vi "SpecPage.vi"(10 "Spec Page Interface":T1, 11 "MetaDataObj in":refnum<class "MetaDataObj.lvclass">) -> (3 "MetaDataObj out":refnum<class "MetaDataObj.lvclass">)   [LabVIEW 2016, in "MeasurementMetaData.lvclass"]
uses:
  MeasurementMetaData.lvclass
  <resource>/dialog/NewProjectWizard/Spec Page Interface.ctl
  <resource>/dialog/NewProjectWizard/MetaDataObj/MetaDataObj.lvclass
  UI References Type Definition.ctl
  C:/Program Files (x86)/National Instruments/LabVIEW 2016/resource/dialog/NewProjectWizard/MetaDataObj/MetaDataObj.lvclass
  MeasurementMetaData.lvclass/MeasurementMetaData.ctl
  <resource>/dialog/NewProjectWizard/MetaDataObj/MetaDataObj.lvclass/MetaDataObj.ctl
  Plugin Settings.ctl
  <resource>/dialog/NewProjectWizard/MetaDataObj/Accessors/Write Project Root.vi
  <resource>/dialog/NewProjectWizard/MetaDataObj/Accessors/Write Project Name.vi
  <resource>/dialog/NewProjectWizard/MetaDataObj/Accessors/Write File Prefix.vi
panel:
  in  "Project Name":string
  in  "Project Root":path
  in  "Measurement Name":string="New Measurement"
  in  "Acquisition Mode":enum16{"Continuous", "Single-Shot"}(ring)=enum."Single-Shot"
  in  "PSU?":bool
  in  "FGEN?":bool
  in  "Scope?":bool
  in  "DMM?":bool
  in  "Override Close Method":bool
  in  "Override Measure Method":bool
  in  "Override Configure Method":bool
  in  "Generate Custom Results Object":bool
  # "Select Methods to Override"
  # "Select Required Hardware"
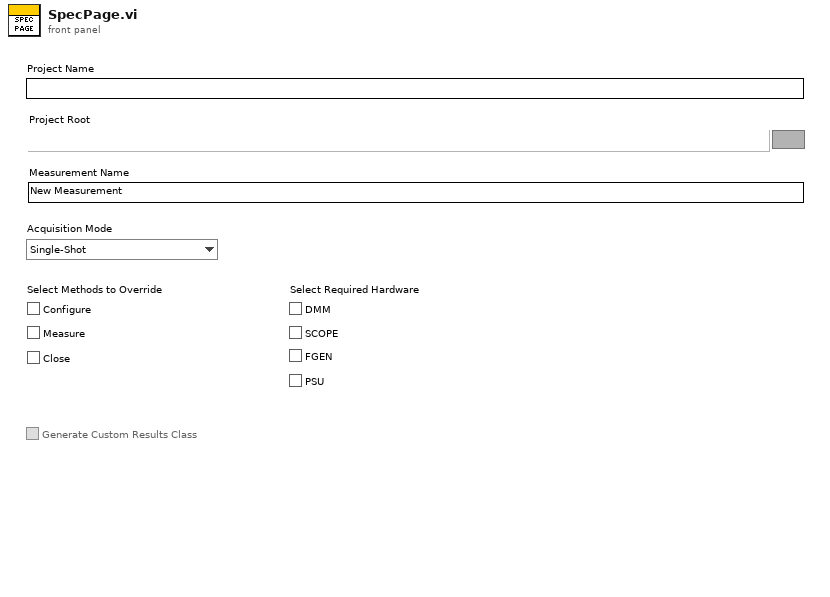
[diagram p1: front panel]
types:
  T1 = typedef "Spec Page Interface.ctl" = cluster{"\"Tab Forward To\" Refnum":refnum<vi>, "\"Tab Backward To\" Refnum":refnum<vi>, "Errors":refnum<user-event>, "Quit":refnum<user-event>}
  T2 = typedef "MeasurementMetaData.lvclass/UI References Type Definition.ctl" = cluster{"Measurement Name":refnum<vi>, "Project Name":refnum<vi>, "Project Root":refnum<vi>, "PSU?":refnum<vi>, "FGEN?":refnum<vi>, "Scope?":refnum<vi>, "DMM?":refnum<vi>, "Override Close Method":refnum<vi>, "Override Measure Method":refnum<vi>, "Generate Custom Results Object":refnum<vi>, "Override Configure Method":refnum<vi>, "Acquisition Mode":refnum<vi>}
  T3 = typedef "MeasurementMetaData.lvclass/Plugin Settings.ctl" = cluster{"Override Configure Method":bool, "Generate Custom Results Object":bool, "Override Measure Method":bool, "Override Close Method":bool, "Scope?":bool, "DMM?":bool, "FGEN?":bool, "PSU?":bool, "Acquisition Mode":enum16{"Continuous", "Single-Shot"}}
  T4 = enum8{"Enabled", "Disabled", "Disabled and Grayed Out"}
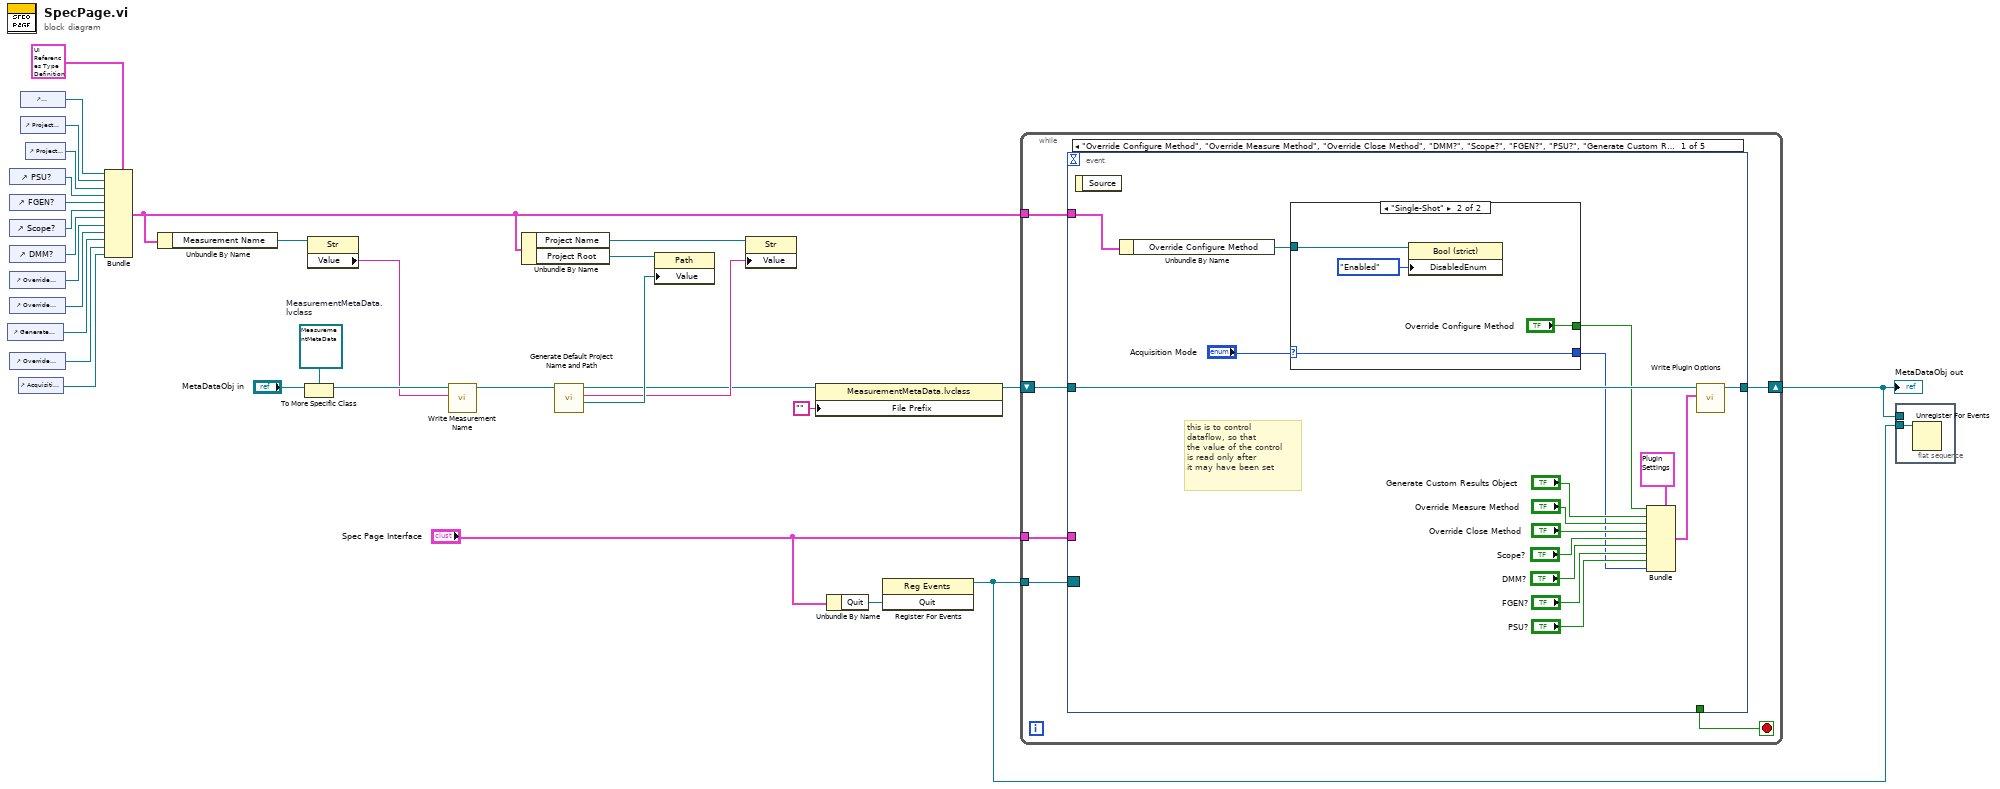
[diagram p0: block diagram]
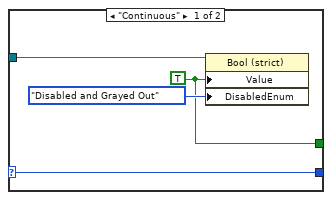
[diagram p2: hidden frame]
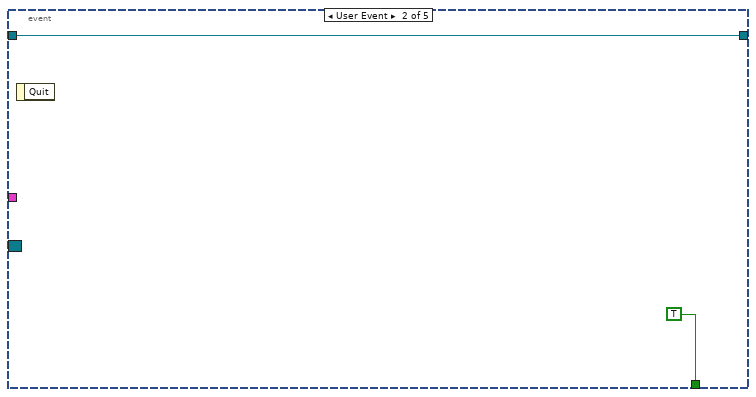
[diagram p3: hidden frame]
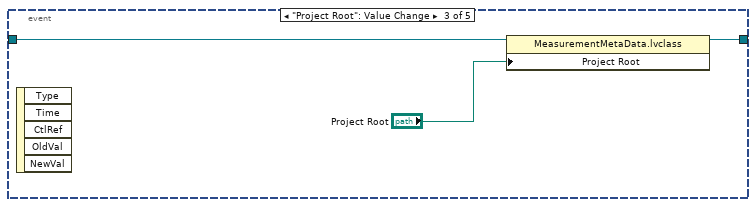
[diagram p4: hidden frame]
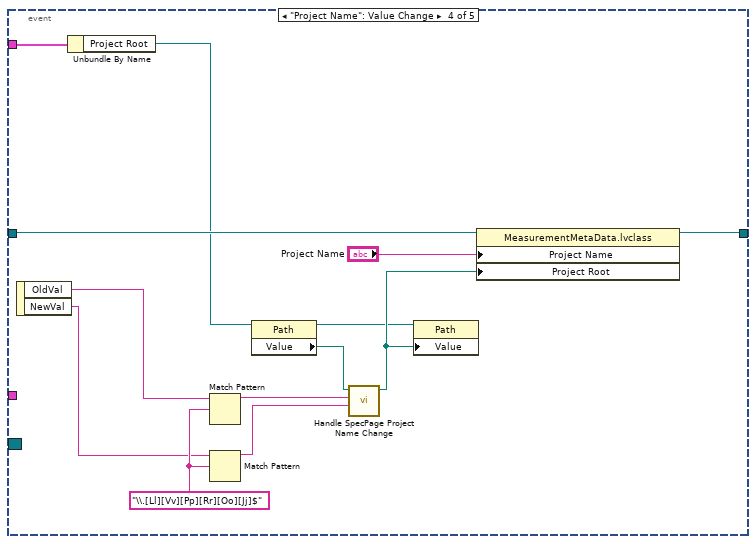
[diagram p5: hidden frame]
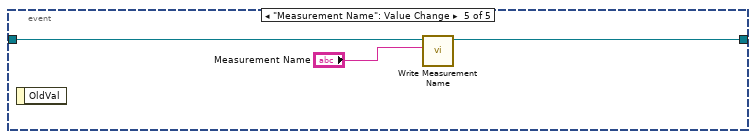
[diagram p6: hidden frame]
diagram:
  w17 = refnum<class "MeasurementMetaData.lvclass"> refnum  # MeasurementMetaData.lvclass
  n1 = control-ref of="Generate Custom Results Object"() -> (w3:refnum<vi>)
  n2 = control-ref of="PSU?"() -> (w25:refnum<vi>)
  n3 = control-ref of="FGEN?"() -> (w24:refnum<vi>)
  n4 = control-ref of="Scope?"() -> (w23:refnum<vi>)
  n5 = control-ref of="DMM?"() -> (w22:refnum<vi>)
  n6 = control-ref of="Override Close Method"() -> (w21:refnum<vi>)
  n7 = control-ref of="Override Measure Method"() -> (w20:refnum<vi>)
  n8 = control-ref of="Override Configure Method"() -> (w1:refnum<vi>)
  n9 = control-ref of="Acquisition Mode"() -> (w2:refnum<vi>)
  n10 = control-ref of="Measurement Name"() -> (w28:refnum<vi>)
  n11 = control-ref of="Project Name"() -> (w27:refnum<vi>)
  n12 = control-ref of="Project Root"() -> (w26:refnum<vi>)
  n13 = Bundle(cluster=T2 {"Measurement Name"=refnum, "Project Name"=refnum, "Project Root"=refnum, "PSU?"=refnum, "FGEN?"=refnum, "Scope?"=refnum, "DMM?"=refnum, "Override Close Method"=refnum, "Override Measure Method"=refnum, "Generate Custom Results Object"=refnum, "Override Configure Method"=refnum, "Acquisition Mode"=refnum} ("output cluster"), "Measurement Name"=w28, "Project Name"=w27, "Project Root"=w26, "PSU?"=w25, "FGEN?"=w24, "Scope?"=w23, "DMM?"=w22, "Override Close Method"=w21, "Override Measure Method"=w20, "Generate Custom Results Object"=w3, "Override Configure Method"=w1, "Acquisition Mode"=w2) -> (w7:T2)
  n14 = Unbundle By Name(w7) -> ("Measurement Name"=w6:refnum<vi>)
  n15 = To More Specific Class(target class=w17, reference="MetaDataObj in") -> (specific class reference=w16:refnum<class "MeasurementMetaData.lvclass">)  [unwired: 1 in, 1 out]
  n16 = property class="Str"(reference=w6) -> ("Value"=w5:string)  [unwired: 1 in, 2 out]
  n17 = call "Write Measurement Name.vi"("Measurement Name"=w5, "MeasurementMetaData in"=w16) -> ("MeasurementMetaData out"=w15:refnum<class "MeasurementMetaData.lvclass">)  [unwired: 8 in, 1 out]
  n18 = Unbundle By Name(w7) -> ("Project Name"=w11:refnum<vi>, "Project Root"=w13:refnum<vi>)
  n19 = call <resource>:"Generate Default Project Name and Path.vi"("DNL_MetaDataObj in"=w15) -> ("Project Root"=w12:path, "Project Name"=w10:string, "DNL_MetaDataObj out"=w4:refnum<class "MeasurementMetaData.lvclass">)  [unwired: 8 in]
  n20 = property class="Path"(reference=w13, "Value"=w12) -> ()  [unwired: 1 in, 2 out]
  n21 = property class="Str"(reference=w11, "Value"=w10) -> ()  [unwired: 1 in, 2 out]
  n22 = property class="MeasurementMetaData.lvclass"(reference=w4, "File Prefix"="") -> (reference out=w8:refnum<class "MeasurementMetaData.lvclass">)  [unwired: 1 in, 1 out]
  n23 = Unbundle By Name("Spec Page Interface") -> ("Quit"=w14:refnum<user-event>)
  n24 = register-events(w14) -> (reference out=w31:refnum<event-registration>)  [unwired: 2 in, 1 out]
  n25 = while {
    tunnel: w31 -> [w35]
    tunnel: w7 -> [w33]
    tunnel: "Spec Page Interface" -> [w32]
    shift-right: [w36] -> w29
    shift-left: w8 -> [w37]
    stop <- w34 stop-if-true
    n26 = event shown="[0] \"Override Configure Method\", \"Override Measure Method\", \"Override Close Method\", \"DMM?\", \"Scope?\", \"FGEN?\", \"PSU?\", \"Generate Custom Results Object\", \"Acquisition Mode\": Value Change" {
      selector: w35 -> [_ _ _ _ _]
      dyn-events: _ -> [_ _ _ _ _]
      timeout: _ -> [_ _ _ _ _]
      tunnel: w37 -> [w49 w62 w65 w79 w81]
      tunnel: [w48 w62 w66 w68 w80] -> w36
      tunnel: [_ TRUE _ _ _] -> w34
      tunnel: w33 -> [w42 _ _ w73 _]
      tunnel: w32 -> [_ _ _ _ _]
      event "Override Configure Method", "Override Measure Method", "Override Close Method", "DMM?", "Scope?", "FGEN?", "PSU?", "Generate Custom Results Object", "Acquisition Mode": Value Change {
        # "this is to control\ndataflow, so that\nthe value of the control\nis read only after\nit may have been set"
        n27 = event-data() -> ()  [unwired: 1 in, 1 out]
        n28 = Unbundle By Name(w42) -> ("Override Configure Method"=w41:refnum<vi>)
        n29 = case shown="\"Single-Shot\"" "Acquisition Mode" {
          selector: "Acquisition Mode" -> [w57 w61]
          tunnel: w41 -> [w56 w60]
          tunnel: [w57 w61] -> w39
          tunnel: [w54 "Override Configure Method"] -> w38
          frame "Continuous" {
            w54 = TRUE ("Value")
            n30 = property class="Bool (strict)"(reference=w56, "Value"=w54, "DisabledEnum"=T4."Disabled and Grayed Out" ("Disabled")) -> ()  [unwired: 1 in, 2 out]
          }
          frame "Single-Shot" {
            n31 = property class="Bool (strict)"(reference=w60, "DisabledEnum"=T4."Enabled" ("Disabled")) -> ()  [unwired: 1 in, 2 out]
          }
        }
        n32 = Bundle(cluster=T3 {"Override Configure Method"=FALSE, "Generate Custom Results Object"=FALSE, "Override Measure Method"=FALSE, "Override Close Method"=FALSE, "Scope?"=FALSE, "DMM?"=FALSE, "FGEN?"=FALSE, "PSU?"=FALSE, "Acquisition Mode"=enum."Continuous"} ("Plugin Options"), "Override Configure Method"=w38, "Generate Custom Results Object"="Generate Custom Results Object", "Override Measure Method"="Override Measure Method", "Override Close Method"="Override Close Method", "Scope?"="Scope?", "DMM?"="DMM?", "FGEN?"="FGEN?", "PSU?"="PSU?", "Acquisition Mode"=w39) -> (w50:T3)
        n33 = call "Write Plugin Options.vi"("Plugin Options"=w50, "MeasurementMetaData in"=w49) -> ("MeasurementMetaData out"=w48:refnum<class "MeasurementMetaData.lvclass">)  [unwired: 8 in, 1 out]
      }
      event User Event {
        n34 = event-data() -> ()  [unwired: 1 in, 1 out]
      }
      event "Project Root": Value Change {
        n35 = event-data() -> ()  [unwired: 1 in, 5 out]
        n36 = property class="MeasurementMetaData.lvclass"(reference=w65, "Project Root"="Project Root") -> (reference out=w66:refnum<class "MeasurementMetaData.lvclass">)  [unwired: 1 in, 1 out]
      }
      event "Project Name": Value Change {
        w78 = "\\.[Ll][Vv][Pp][Rr][Oo][Jj]$" ("regular expression")
        n37 = event-data() -> ("OldVal"=w77:string, "NewVal"=w76:string)  [unwired: 1 in]
        n38 = Unbundle By Name(w73) -> ("Project Root"=w72:refnum<vi>)
        n39 = Match Pattern(string=w77, regular expression=w78) -> (before substring=w74:string)  [unwired: 1 in, 3 out]
        n40 = Match Pattern(string=w76, regular expression=w78) -> (before substring=w75:string)  [unwired: 1 in, 3 out]
        n41 = property class="Path"(reference=w72) -> (reference out=w69:refnum<vi>, "Value"=w71:path)  [unwired: 1 in, 1 out]
        n42 = call <resource>:"Handle SpecPage Project Name Change.vi"("Project Name New Value"=w75, "Project Name Old Value"=w74, "Project Root in"=w71) -> ("Project Root out"=w70:path)  [unwired: 8 in]
        n43 = property class="Path"(reference=w69, "Value"=w70) -> ()  [unwired: 1 in, 2 out]
        n44 = property class="MeasurementMetaData.lvclass"(reference=w79, "Project Name"="Project Name", "Project Root"=w70) -> (reference out=w68:refnum<class "MeasurementMetaData.lvclass">)  [unwired: 1 in, 1 out]
      }
      event "Measurement Name": Value Change {
        n45 = event-data() -> ()  [unwired: 1 in, 1 out]
        n46 = call "Write Measurement Name.vi"("Measurement Name"="Measurement Name", "MeasurementMetaData in"=w81) -> ("MeasurementMetaData out"=w80:refnum<class "MeasurementMetaData.lvclass">)  [unwired: 8 in, 1 out]
      }
    }
  }
  "MetaDataObj out" <- w29
  n47 = flat-sequence {
    tunnel: w31 -> [w83]
    tunnel: w29 -> [_]
    frame #0 {
      n48 = Unregister For Events(event registration refnum=w83) -> ()  [unwired: 1 in, 1 out]
    }
  }
